vi "Init.vi"(8 "error in (no error)":errorcluster, 11 "Simulated in":refnum<class "Simulated.lvclass">) -> (0 "error out":errorcluster, 3 "Simulated out":refnum<class "Simulated.lvclass">)   [LabVIEW 2016, in "Simulated.lvclass"]
uses:
  Simulated.lvclass
  Parent/Hardware.lvclass
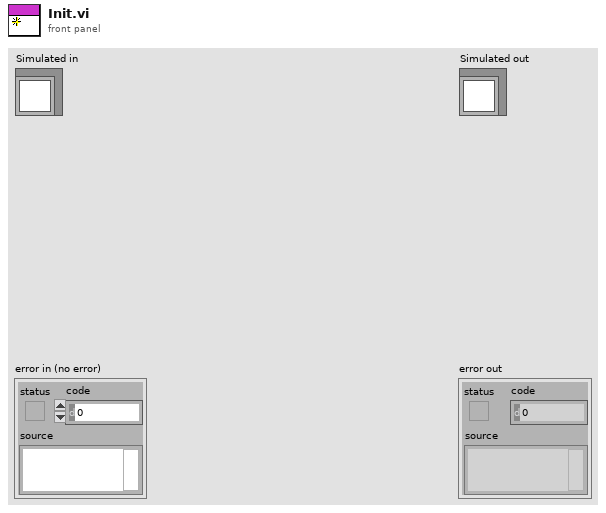
[diagram p1: front panel]
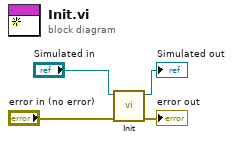
[diagram p0: block diagram]
diagram:
  n1 = call-parent "Init.vi"("error in (no error)"="error in (no error)", "Hardware in"="Simulated in") -> ("error out"=→"error out":errorcluster, "Hardware out"=→"Simulated out":refnum<class "Simulated.lvclass">)  [unwired: 8 in]
